vi "Save Limit Test Template.vi"(8 "error in (no error)":errorcluster, 10 "Template Source (0:Channel 1)":i32(ring) items=["First Template Source", "Second Template Source", "Single Template Source"], 11 "VISA resource name":refnum<visa-resource-name>) -> (0 "error out":errorcluster, 3 "VISA resource name out":refnum<visa-resource-name>)   [LabVIEW 2017, in "Tektronix TDS 200 1000 2000 Series.lvlib"]
doc: "This VI saves the template source data information.\n\n<b>Note(s):</b>\n1. This VI is only applicable for TBS1000B series models.\n2. This VI does not check the instrument status."
uses:
  Tektronix TDS 200 1000 2000 Series.lvlib
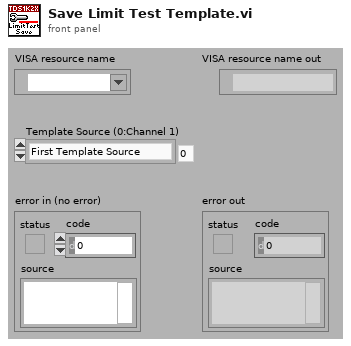
[diagram p1: front panel]
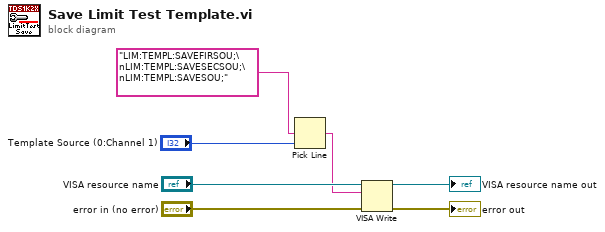
[diagram p0: block diagram]
diagram:
  n1 = Pick Line(multi-line string="LIM:TEMPL:SAVEFIRSOU;\nLIM:TEMPL:SAVESECSOU;\nLIM:TEMPL:SAVESOU;", line index="Template Source (0:Channel 1)") -> (output string=w3:string)  [unwired: 1 out]
  n2 = VISA Write(VISA resource name="VISA resource name", write buffer=w3, error in (no error)="error in (no error)") -> (VISA resource name out=→"VISA resource name out":refnum<visa-resource-name>, error out=→"error out":errorcluster)  [unwired: 1 out]
